vi "create_image_name_file.vi"(8 "error in (no error)":errorcluster, 9 "target format":T1, 10 "target image path":path, 11 "Image in":refnum<class "Image.lvclass">) -> (0 "error out":errorcluster, 2 "file name":string, 3 "Image out":refnum<class "Image.lvclass">)   [LabVIEW 2010]
uses:
  Image.lvclass
  ImageCollection/target_format_enum.ctl
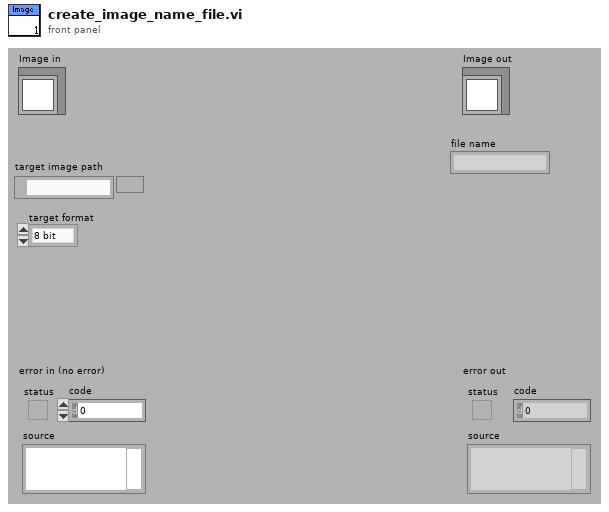
[diagram p1: front panel]
types:
  T1 = typedef "ImageCollection.lvclass/target_format_enum.ctl" = enum16{"8 bit", "16 bit", "32 bit"}
  T2 = enum16{"open", "replace", "create", "open or create", "replace or create", "replace or create with confirmation"}
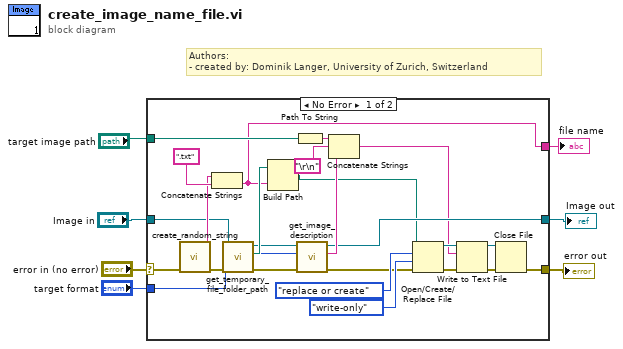
[diagram p0: block diagram]
diagram:
  # "Authors: \n- created by: Dominik Langer, University of Zurich, Switzerland"
  n1 = case shown="No Error" "error in (no error)" {
    selector: "error in (no error)" -> [w32 w34]
    tunnel: [w12 w34] -> w6
    tunnel: [w20 w33] -> w4
    tunnel: "Image in" -> [w27 w33]
    tunnel: "target image path" -> [w24 _]
    tunnel: [w9 _] -> w2
    tunnel: "target format" -> [w8 _]
    frame No Error {
      n2 = call "create_random_string.vi"("error in (no error)"=w32) -> ("error out"=w31:errorcluster, "random string"=w29:string)  [unwired: 1 in, 8 out]
      n3 = Concatenate Strings(w29, ".txt" ("string")) -> (w9:string)
      n4 = call-dynamic "get_temporary_file_folder_path.vi"("error in (no error)"=w31, "Image in"=w27) -> ("error out"=w23:errorcluster, "temp file folder"=w28:path, "Image out"=w21:refnum<class "Image.lvclass">)  [unwired: 7 out]
      n5 = Build Path(base path=w28, name or relative path=w9) -> (appended path=w11:path)
      n6 = Path To String(path=w24) -> (string=w25:string)
      n7 = call "get_image_description.vi"("error in (no error)"=w23, 10:w8, "Image in"=w21) -> ("error out"=w13:errorcluster, "image description"=w22:string, "Image out"=w20:refnum<class "Image.lvclass">)  [unwired: 6 out]
      n8 = Concatenate Strings(w25, "\r\n", w22) -> (w10:string)
      n9 = Open/Create/Replace File(file path (use dialog)=w11, error in=w13, operation (0:open)=T2."replace or create", access (0:read/write)=enum16{"read/write", "read-only", "write-only"}."write-only") -> (refnum out=w14:refnum<file>, error out=w15:errorcluster)  [unwired: 3 out]
      n10 = Write to Text File(file (use dialog)=w14, text=w10, error in=w15) -> (refnum out=w16:refnum<file>, error out=w17:errorcluster)  [unwired: 2 out]
      n11 = Close File(refnum=w16, error in=w17) -> (error out=w12:errorcluster)  [unwired: 1 out]
    }
    frame Error {
    }
  }
  "error out" <- w6
  "Image out" <- w4
  "file name" <- w2
